vi "main.vi"() -> ()   [LabVIEW 2020]
uses:
  <vilib>/express/express analysis/Spectral/Block/exnSpectralBlock spectral measurements peak poly.vi
  <vilib>/express/express analysis/Spectral/Block/exnSpectralBlock spectral measurements peak DDT.vi
  <vilib>/express/express analysis/Spectral/XNode/ExpressSpectralMeasurementsBlockNode.xnode
panel:
  in  "Tab Control":enum32{"Generador", "Procesador"}(tab)
  in  "Tecla_D":bool
  in  "Tecla_#":bool
  in  "Tecla_0":bool
  in  "Tecla_*":bool
  in  "Tecla_C":bool
  in  "Tecla_9":bool
  in  "Tecla_8":bool
  in  "Tecla_7":bool
  in  "Tecla_B":bool
  in  "Tecla_6":bool
  in  "Tecla_5":bool
  in  "Tecla_4":bool
  in  "Tecla_A":bool
  in  "Tecla_3":bool
  in  "Tecla_2":bool
  in  "Tecla_1":bool
  out "Frecuencia_Mayor":dbl
  out "Frecuencia_Menor":dbl
  out "String":string
  out "Acquire_Sound":dynamicdata(graph) caption="Data"
  out "Spectral_Measurements":dynamicdata(graph)
  in  "stop":bool
  # "GENERADOR / PROCESADOR DE SEÑALES DTMF"
  # "Escuchando..."
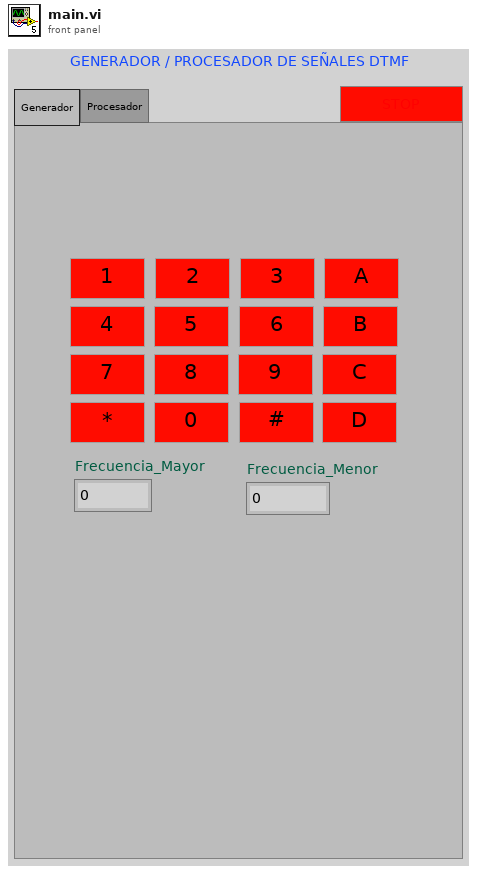
[diagram p1: front panel]
types:
  T1 = enum16{"Inicio", "Validar_Tecla_Pulsada", "Reproducir_Sonido", "Validar_Frecuencias", "Identificar_Tecla"}
  T2 = cluster{"averaging mode":u16, "weighting mode":u16, "number of averages":u32}
  T3 = cluster{"dB On (F)":bool, "unwrap phase (F)":bool, "convert to degree (F)":bool}
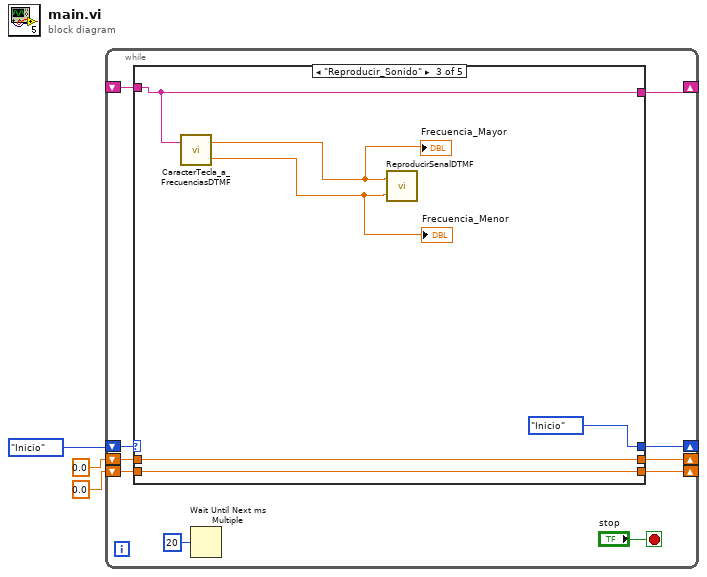
[diagram p0: block diagram]
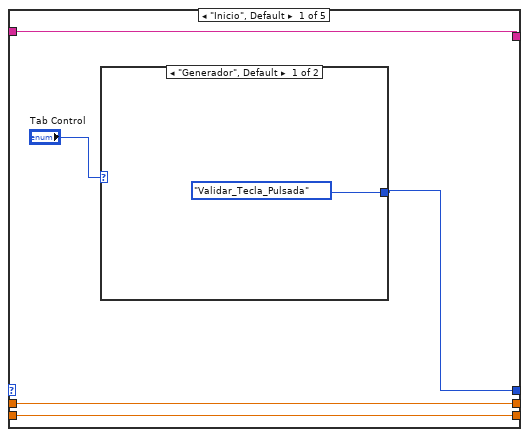
[diagram p2: hidden frame]
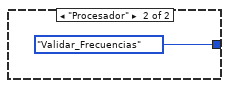
[diagram p3: hidden frame]
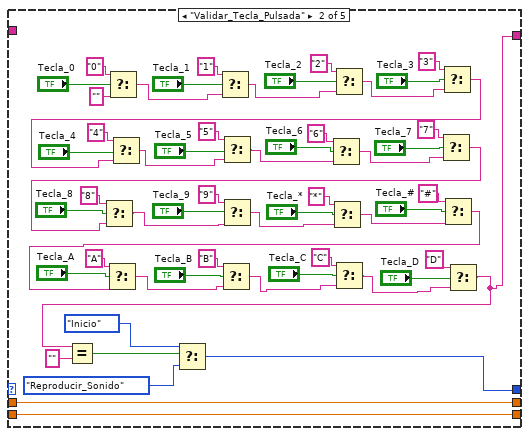
[diagram p4: hidden frame]
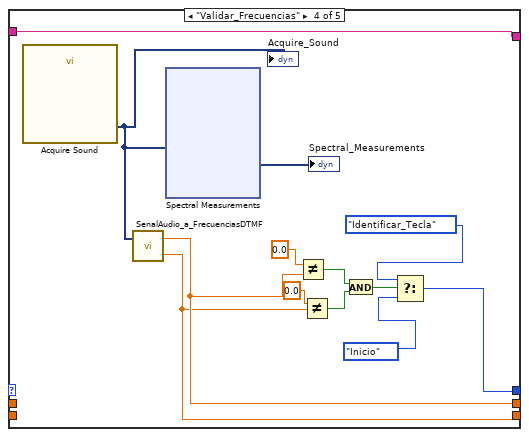
[diagram p5: hidden frame]
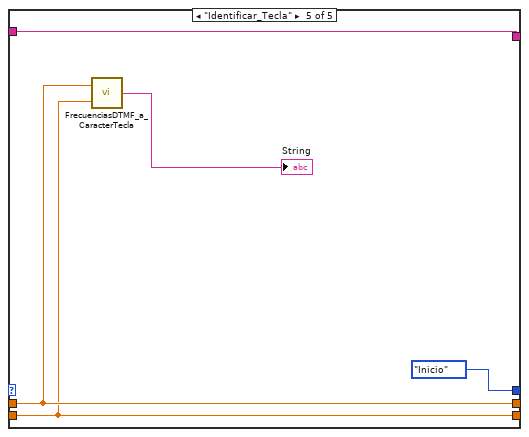
[diagram p6: hidden frame]
diagram:
  n1 = while {
    shift-right: [w10] -> _
    shift-left: T1."Inicio" ("Estados") -> [w11]
    shift-right: [w9] -> _
    shift-left: _ -> [w8]
    shift-right: [w7] -> _
    shift-left: 0.0 ("Max_Frecuencia") -> [w5]
    shift-right: [w6] -> _
    shift-left: 0.0 ("Min_Frecuencia") -> [w4]
    stop <- "stop" stop-if-true
    n2 = case shown="\"Reproducir_Sonido\"" w11 {
      tunnel: [w14 w24 T1."Inicio" ("Estados") w85 T1."Inicio" ("Estados")] -> w10
      tunnel: [w18 w23 w81 w95 w109] -> w9
      tunnel: w8 -> [w18 _ w81 w95 w109]
      tunnel: [w17 w22 w80 w84 w108] -> w7
      tunnel: [w16 w21 w79 w83 w107] -> w6
      tunnel: w5 -> [w17 w22 w80 _ w108]
      tunnel: w4 -> [w16 w21 w79 _ w107]
      frame "Inicio", Default {
        n3 = case shown="\"Generador\", Default" "Tab Control" {
          tunnel: [T1."Validar_Tecla_Pulsada" ("Estados") T1."Validar_Frecuencias" ("Estados")] -> w14
          frame "Generador", Default {
          }
          frame "Procesador" {
          }
        }
      }
      frame "Validar_Tecla_Pulsada" {
        n4 = Select(t="0", s="Tecla_0", f="") -> (s? t:f=w74:string)
        n5 = Select(t="1", s="Tecla_1", f=w74) -> (s? t:f=w73:string)
        n6 = Select(t="2", s="Tecla_2", f=w73) -> (s? t:f=w71:string)
        n7 = Select(t="3", s="Tecla_3", f=w71) -> (s? t:f=w68:string)
        n8 = Select(t="4", s="Tecla_4", f=w68) -> (s? t:f=w66:string)
        n9 = Select(t="5", s="Tecla_5", f=w66) -> (s? t:f=w64:string)
        n10 = Select(t="6", s="Tecla_6", f=w64) -> (s? t:f=w62:string)
        n11 = Select(t="7", s="Tecla_7", f=w62) -> (s? t:f=w60:string)
        n12 = Select(t="8", s="Tecla_8", f=w60) -> (s? t:f=w58:string)
        n13 = Select(t="9", s="Tecla_9", f=w58) -> (s? t:f=w56:string)
        n14 = Select(t="*", s="Tecla_*", f=w56) -> (s? t:f=w54:string)
        n15 = Select(t="#", s="Tecla_#", f=w54) -> (s? t:f=w52:string)
        n16 = Select(t="A", s="Tecla_A", f=w52) -> (s? t:f=w50:string)
        n17 = Select(t="B", s="Tecla_B", f=w50) -> (s? t:f=w49:string)
        n18 = Select(t="C", s="Tecla_C", f=w49) -> (s? t:f=w29:string)
        n19 = Select(t="D", s="Tecla_D", f=w29) -> (s? t:f=w23:string)
        n20 = Equal?(x=w23, y="") -> (x = y?=w26:bool)
        n21 = Select(t=T1."Inicio" ("Estados"), s=w26, f=T1."Reproducir_Sonido" ("Estados")) -> (s? t:f=w24:T1)
      }
      frame "Reproducir_Sonido" {
        n22 = call "CaracterTecla_a_FrecuenciasDTMF.vi"("Caracter_Tecla"=w81) -> ("Min_Frecuencia"=w77:dbl, "Max_Frecuencia"=w78:dbl)  [unwired: 1 in]
        "Frecuencia_Mayor" <- w78
        "Frecuencia_Menor" <- w77
        n23 = call "ReproducirSenalDTMF.vi"("Min_Frecuencia"=w77, "Max_Frecuencia"=w78) -> ()  [unwired: 2 in]
      }
      frame "Validar_Frecuencias" {
        n24 = call "Acquire Sound"() -> ("Data"=w93:dynamicdata)  [unwired: 18 in, 1 out]
        "Acquire_Sound" <- w93
        n25 = call "SenalAudio_a_FrecuenciasDTMF.vi"("time signal in"=w93) -> ("Min_Frecuencia"=w83:dbl, "Max_Frecuencia"=w84:dbl)  [unwired: 1 in]
        n26 = xnode "Spectral Measurements"("Signals"=w93) -> ("FFT - (Peak)"=→"Spectral_Measurements":dynamicdata)  [unwired: 1 in, 2 out]
        n27 = Not Equal?(x=0.0, y=w84) -> (x != y?=w89:bool)
        n28 = Not Equal?(x=0.0, y=w83) -> (x != y?=w90:bool)
        n29 = And(x=w89, y=w90) -> (x .and. y?=w88:bool)
        n30 = Select(t=T1."Identificar_Tecla" ("Estados"), s=w88, f=T1."Inicio" ("Estados")) -> (s? t:f=w85:T1)
      }
      frame "Identificar_Tecla" {
        n31 = call "FrecuenciasDTMF_a_CaracterTecla.vi"("Min_Frecuencia"=w107, "Max_Frecuencia"=w108) -> ("Caracter_Tecla"=→"String":string)
      }
    }
    n32 = Wait Until Next ms Multiple(millisecond multiple=u32 20) -> ()  [unwired: 1 out]
  }
